vi "set engine advansed setup.vi"(8 "error in (no error)":errorcluster, 10 "engine_advansed_setup":T1, 11 "id":i32) -> (0 "error out":errorcluster, 3 "function return":i32)   [LabVIEW 2012, in "libximc.lvlib"]
doc: "result_t XIMC_API set_engine_advansed_setup (device_t id, const engine_advansed_setup_t* engine_advansed_setup);"
uses:
  libximc.lvlib
  libximc.dll
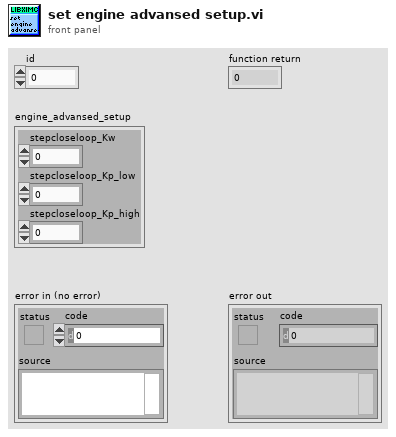
[diagram p1: front panel]
types:
  T1 = cluster{"stepcloseloop_Kw":u32, "stepcloseloop_Kp_low":u32, "stepcloseloop_Kp_high":u32}
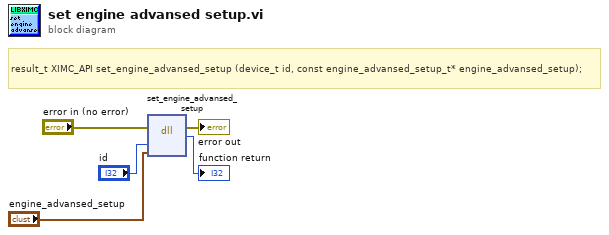
[diagram p0: block diagram]
diagram:
  # "result_t XIMC_API set_engine_advansed_setup (device_t id, const engine_advansed_setup_t* engine_advansed_setup);"
  n1 = dll-call lib="E:/labview-2.12.1-Labview_12.0/ximcLVx32/libximc.*" fn="set_engine_advansed_setup"(error in="error in (no error)", "id"="id", "engine_advansed_setup"="engine_advansed_setup") -> (error out=→"error out":errorcluster, →"function return":i32)  [unwired: 4 in, 1 out]
